vi "stimulate_and_record.vi"(3 "SSH password":string, 4 "Transfer and Run Date Folder After Experiment":bool, 5 "SSH user name":string, 6 "Tags":string, 7 "Frames":i32, 8 "Convert Power to Voltage":bool, 9 "voltages/power":dbl[](array[numeric]), 10 "parameters":string[](array[string]), 11 "parameters headers":string[](array[string])) -> ()   [LabVIEW 2014]
uses:
  <vilib>/userdefined/High Color/IMAQdx.ctl
  <vilib>/Utility/file.llb/Write To Spreadsheet File (string).vi
  <vilib>/Utility/file.llb/Read From Spreadsheet File (string).vi
  <vilib>/Utility/file.llb/Write To Spreadsheet File (DBL).vi
panel:
  out "Error":string
  out "Save Directory":path
  out "Buffer Number Out":u32
  out "Image":T1(plugin-control)
  in  "stop":bool
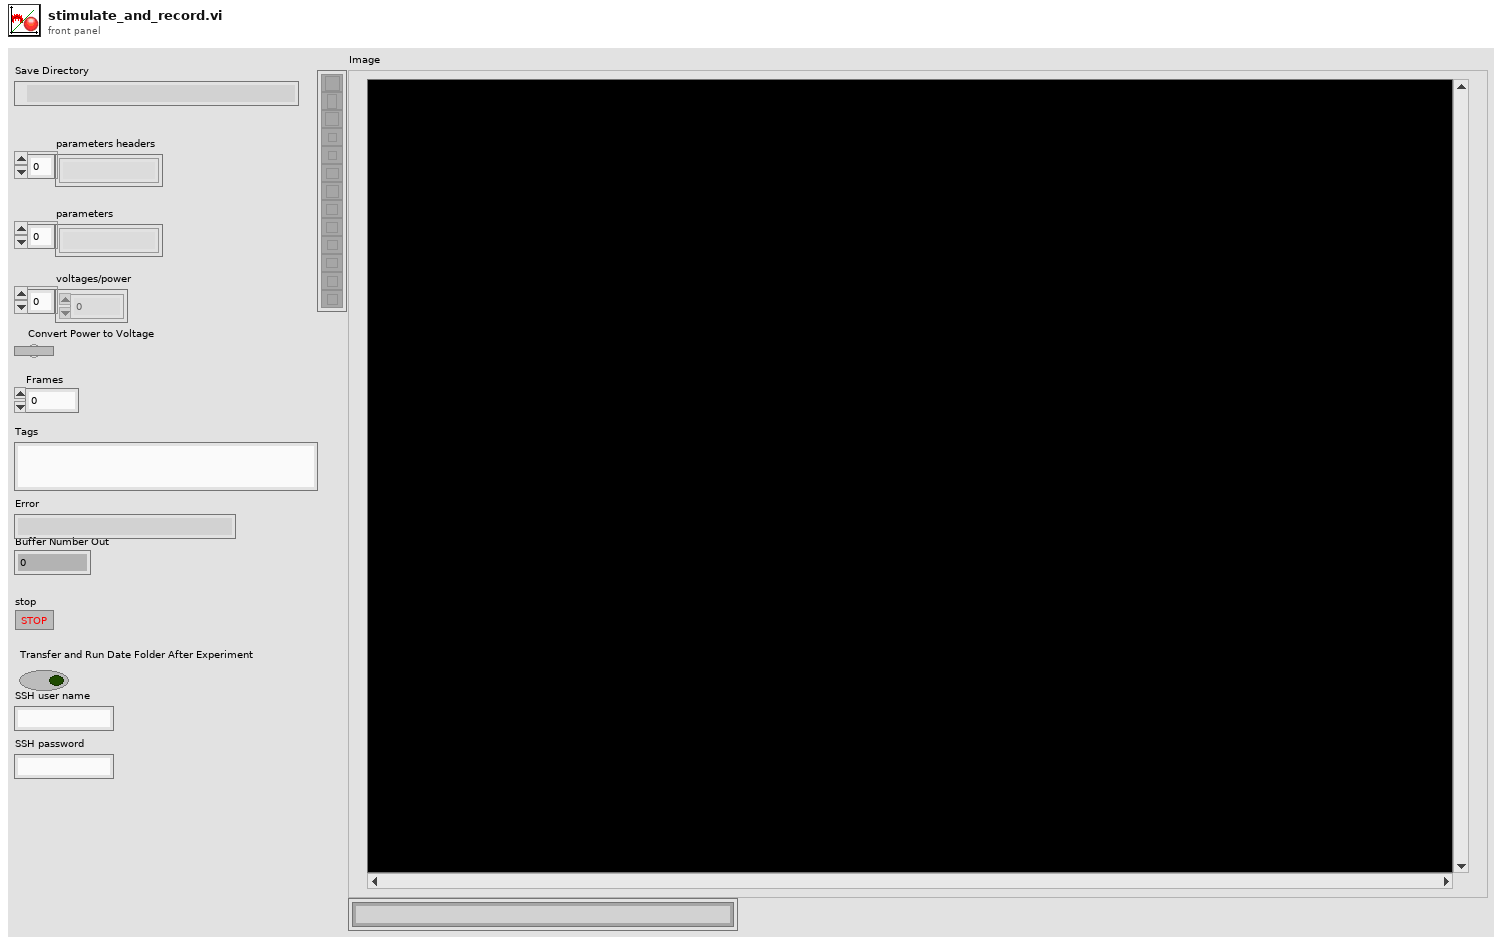
[diagram p1: front panel]
types:
  T1 = typedef "IMAQ Image.ctl" = refnum<image>
  T2 = typedef "IMAQdx.ctl" = refnum<k21>
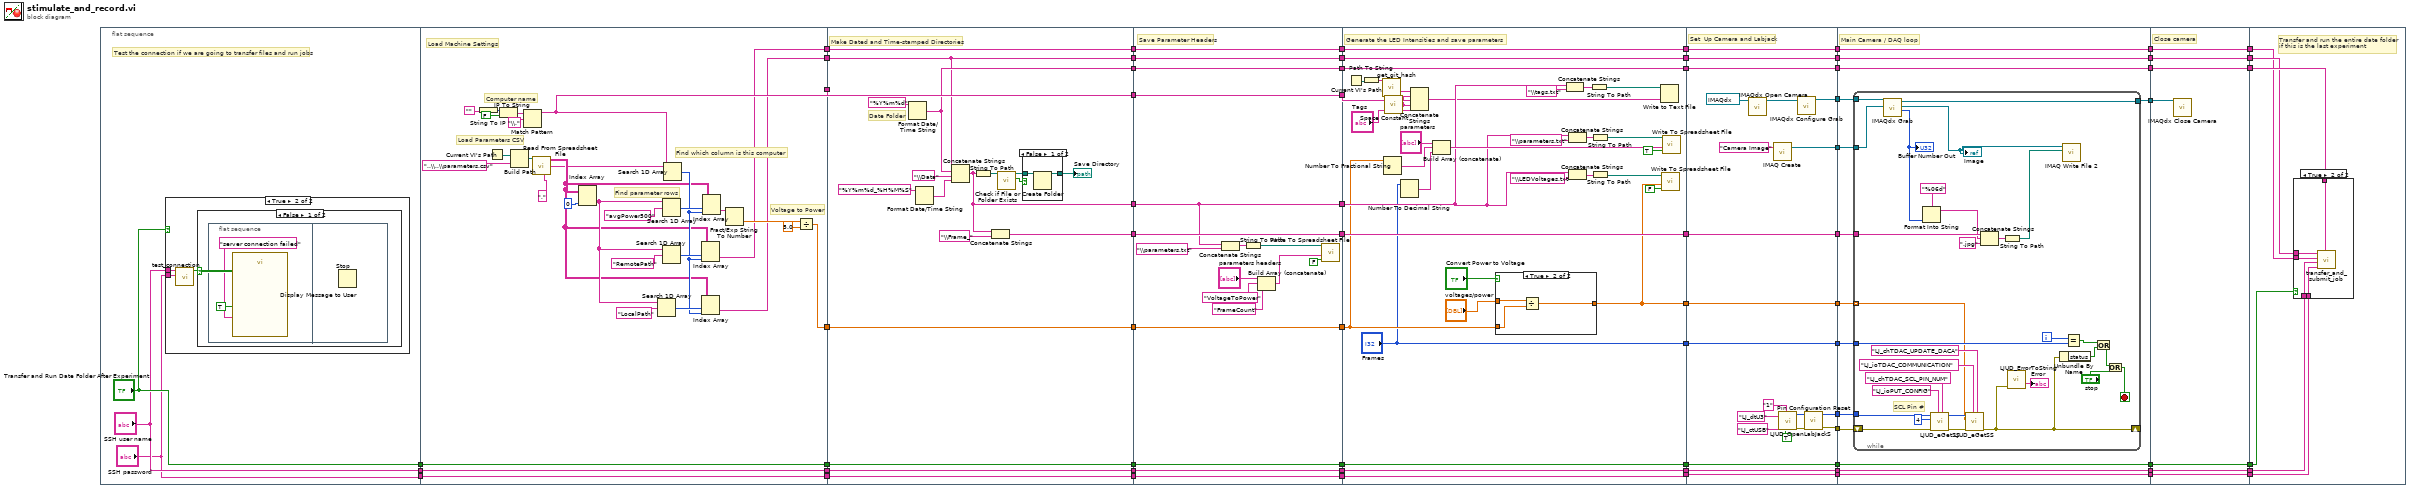
[diagram p0: block diagram]
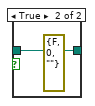
[diagram p4: hidden frame]
diagram:
  n1 = flat-sequence {
    tunnel: ["Transfer and Run Date Folder After Experiment"] -> w24
    tunnel: ["SSH user name"] -> w23
    tunnel: ["SSH password"] -> w22
    tunnel: [w95] -> w54
    tunnel: [w94] -> w53
    tunnel: [w83] -> w44
    tunnel: [w82] -> w43
    tunnel: w24 -> [w76]
    tunnel: w23 -> [w75]
    tunnel: w22 -> [w74]
    tunnel: [w76] -> w15
    tunnel: [w75] -> w8
    tunnel: [w74] -> w7
    tunnel: [w122] -> w38
    tunnel: [w121] -> w36
    tunnel: [w120] -> w34
    tunnel: [w119] -> w32
    tunnel: [w118] -> w30
    tunnel: [w117] -> w28
    tunnel: [w116] -> w26
    tunnel: w43 -> [w116]
    tunnel: w44 -> [w117]
    tunnel: w53 -> [w119]
    tunnel: w54 -> [w120]
    tunnel: [w106] -> w16
    tunnel: w15 -> [w106]
    tunnel: [w105] -> w9
    tunnel: w8 -> [w105]
    tunnel: w7 -> [w104]
    tunnel: [w104] -> w6
    tunnel: w38 -> [w143]
    tunnel: [w143] -> w37
    tunnel: w36 -> [w129]
    tunnel: [w129] -> w35
    tunnel: w34 -> [w142]
    tunnel: [w142] -> w33
    tunnel: w32 -> [w141]
    tunnel: [w141] -> w31
    tunnel: w30 -> [w140]
    tunnel: [w140] -> w29
    tunnel: w28 -> [w139]
    tunnel: [w139] -> w27
    tunnel: w26 -> [w138]
    tunnel: [w138] -> w25
    tunnel: [w128] -> w17
    tunnel: w16 -> [w128]
    tunnel: [w127] -> w10
    tunnel: w9 -> [w127]
    tunnel: w6 -> [w126]
    tunnel: [w126] -> w5
    tunnel: w37 -> [w176]
    tunnel: [w176] -> w59
    tunnel: [w156] -> w57
    tunnel: ["Frames"] -> w56
    tunnel: w35 -> [w168]
    tunnel: w33 -> [w152]
    tunnel: w31 -> [w164]
    tunnel: w29 -> [w161]
    tunnel: [w161] -> w49
    tunnel: [w160] -> w45
    tunnel: w27 -> [w160]
    tunnel: [w159] -> w39
    tunnel: w25 -> [w159]
    tunnel: [w150] -> w18
    tunnel: w17 -> [w150]
    tunnel: [w149] -> w11
    tunnel: w10 -> [w149]
    tunnel: w5 -> [w148]
    tunnel: [w148] -> w4
    tunnel: w59 -> [w199]
    tunnel: [w201] -> w65
    tunnel: [w200] -> w64
    tunnel: [w199] -> w63
    tunnel: [w191] -> w61
    tunnel: [w190] -> w60
    tunnel: [w195] -> w58
    tunnel: w57 -> [w195]
    tunnel: w56 -> [w194]
    tunnel: [w194] -> w55
    tunnel: [w188] -> w50
    tunnel: w49 -> [w188]
    tunnel: [w187] -> w46
    tunnel: w45 -> [w187]
    tunnel: [w186] -> w40
    tunnel: w39 -> [w186]
    tunnel: [w185] -> w19
    tunnel: w18 -> [w185]
    tunnel: [w184] -> w12
    tunnel: w11 -> [w184]
    tunnel: w4 -> [w183]
    tunnel: [w183] -> w3
    tunnel: w65 -> [w218]
    tunnel: w64 -> [w217]
    tunnel: w63 -> [w216]
    tunnel: [w215] -> w62
    tunnel: w61 -> [w214]
    tunnel: w60 -> [w213]
    tunnel: w58 -> [w212]
    tunnel: w55 -> [w211]
    tunnel: [w210] -> w51
    tunnel: w50 -> [w210]
    tunnel: [w209] -> w47
    tunnel: w46 -> [w209]
    tunnel: [w208] -> w41
    tunnel: w40 -> [w208]
    tunnel: [w207] -> w20
    tunnel: w19 -> [w207]
    tunnel: [w206] -> w13
    tunnel: w12 -> [w206]
    tunnel: w3 -> [w205]
    tunnel: [w205] -> w2
    tunnel: w62 -> [w255]
    tunnel: [w254] -> w52
    tunnel: w51 -> [w254]
    tunnel: [w253] -> w48
    tunnel: w47 -> [w253]
    tunnel: [w252] -> w42
    tunnel: w41 -> [w252]
    tunnel: [w251] -> w21
    tunnel: w20 -> [w251]
    tunnel: [w250] -> w14
    tunnel: w13 -> [w250]
    tunnel: w2 -> [w249]
    tunnel: [w249] -> w1
    tunnel: w52 -> [w261]
    tunnel: w48 -> [w260]
    tunnel: w42 -> [w259]
    tunnel: w21 -> [w258]
    tunnel: w14 -> [w257]
    tunnel: w1 -> [w256]
    frame #0 {
      # "Test the connection if we are going to transfer files and run jobs"
      n2 = case shown="True" "Transfer and Run Date Folder After Experiment" {
        tunnel: "SSH password" -> [_ w71]
        tunnel: "SSH user name" -> [_ w69]
        frame False {
        }
        frame True {
          n3 = call "test_connection.vi"("Username"=w69, "Password"=w71) -> ("Connection Successful"=w70:bool)  [unwired: 7 in]
          n4 = case shown="False" w70 {
            frame False {
              n5 = flat-sequence {
                frame #0 {
                  n6 = call "Display Message to User"("Enable"=TRUE, "Message"="server connection failed") -> ()  [unwired: 8 in, 2 out]
                }
                frame #1 {
                  n7 = Stop() -> ()  [unwired: 1 in]
                }
              }
            }
            frame True {
            }
          }
        }
      }
    }
    frame #1 {
      # "Find parameter rows"
      # "Find which column is this computer"
      # "Voltage to Power"
      # "Load Parameters CSV"
      # "Computer name"
      # "Load Machine Settings"
      n8 = String To IP(1:"") -> (0:w103:u32)
      n9 = Current VI's Path() -> (path=w98:path)
      n10 = IP To String(1:FALSE, 2:w103) -> (0:w100:string)
      n11 = Build Path(base path=w98, name or relative path="..\\..\\parameters.csv") -> (appended path=w80:path)
      n12 = Match Pattern(string=w100, regular expression="\\.") -> (before substring=w94:string)  [unwired: 1 in, 3 out]
      n13 = call-poly <vilib>:"Read From Spreadsheet File.vi"("delimiter (\\t)"=",", "file path (dialog if empty)"=w80) -> ("first row"=w78:string[], "all rows"=w79:string[][])  [unwired: 5 in, 3 out]
      n14 = Index Array(array=w79, index (col)=0) -> (element=w81:string[])  [unwired: 1 in]
      n15 = Search 1D Array(1D array=w81, element="LocalPath") -> (index of element=w85:i32)  [unwired: 1 in]
      n16 = Search 1D Array(1D array=w81, element="RemotePath") -> (index of element=w89:i32)  [unwired: 1 in]
      n17 = Search 1D Array(1D array=w81, element="avgPower500") -> (index of element=w90:i32)  [unwired: 1 in]
      n18 = Search 1D Array(1D array=w78, element=w94) -> (index of element=w84:i32)  [unwired: 1 in]
      n19 = Index Array(array=w79, index (row)=w89, index (col)=w84) -> (element=w82:string)
      n20 = Index Array(array=w79, index (row)=w85, index (col)=w84) -> (element=w83:string)
      n21 = Index Array(array=w79, index (row)=w90, index (col)=w84) -> (element=w88:string)
      n22 = Fract/Exp String To Number(string=w88) -> (number=w87:dbl)  [unwired: 3 in, 1 out]
      n23 = Divide(x=w87, y=5.0) -> (x/y=w95:dbl)
    }
    frame #2 {
      # "Date Folder"
      # "Make Dated and Time-stamped Directories"
      n24 = Format Date/Time String(time format string (%c)="%Y%m%d") -> (date/time string=w118:string)  [unwired: 2 in]
      n25 = Format Date/Time String(time format string (%c)="%Y%m%d_%H%M%S") -> (date/time string=w110:string)  [unwired: 2 in]
      n26 = Concatenate Strings(w117, w118, "\\Data", w110) -> (w121:string)
      n27 = String To Path(string=w121) -> (path=w109:path)
      n28 = Concatenate Strings(w121, "\\Frame_") -> (w122:string)
      n29 = call <vilib>:"Check if File or Folder Exists.vi"("path"=w109) -> ("file or folder exists?"=w114:bool, "dup path"=w113:path)  [unwired: 8 in, 1 out]
      n30 = case shown="False" w114 {
        tunnel: [w123 w125] -> w108
        tunnel: w113 -> [w124 w125]
        frame False {
          n31 = Create Folder(path (use dialog)=w124) -> (created path=w123:path)  [unwired: 2 in, 2 out]
        }
        frame True {
          (unwired) errorcluster {"status"=FALSE, "code"=0, "source"=""} ("error out")
        }
      }
      "Save Directory" <- w108
    }
    frame #3 {
      # "Save Parameter Headers"
      n32 = Concatenate Strings(w129, "\\parameters.txt") -> (w137:string)
      n33 = String To Path(string=w137) -> (path=w136:path)
      n34 = Build Array (concatenate)("parameters headers", "VoltageToPower", "FrameCount") -> (w133:string[])
      n35 = call-poly <vilib>:"Write To Spreadsheet File.vi"("append to file? (new file:F)"=FALSE, "1D data"=w133, "file path (dialog if empty)"=w136) -> ()  [unwired: 5 in, 1 out]
    }
    frame #4 {
      # "Generate the LED Intensities and save parameters"
      n36 = Current VI's Path() -> (path=w146:path)
      n37 = Path To String(path=w146) -> (string=w147:string)
      n38 = call "get_git_hash.vi"("VI folder"=w147) -> ("github hash"=w144:string)  [unwired: 10 in]
      n39 = Number To Fractional String(number=w152) -> (F-format string=w153:string)  [unwired: 3 in]
      n40 = call <vilib>:"Space Constant.vi"() -> ("String"=w145:string)
      n41 = Number To Decimal String(number="Frames") -> (decimal integer string=w154:string)  [unwired: 1 in]
      n42 = Concatenate Strings(w144, w145, w164, w145, "Tags") -> (w162:string)
      n43 = Build Array (concatenate)("parameters", w153, w154) -> (w169:string[])
      n44 = case shown="True" "Convert Power to Voltage" {
        tunnel: "voltages/power" -> [w179 w182]
        tunnel: [w179 w180] -> w156
        tunnel: w152 -> [_ w181]
        frame False {
        }
        frame True {
          n45 = Divide(x=w182, y=w181) -> (x/y=w180:dbl[])
        }
      }
      n46 = Concatenate Strings(w168, "\\tags.txt") -> (w166:string)
      n47 = Concatenate Strings(w168, "\\LEDVoltages.txt") -> (w178:string)
      n48 = Concatenate Strings(w168, "\\parameters.txt") -> (w173:string)
      n49 = String To Path(string=w166) -> (path=w165:path)
      n50 = String To Path(string=w178) -> (path=w177:path)
      n51 = String To Path(string=w173) -> (path=w172:path)
      n52 = Write to Text File(file (use dialog)=w165, text=w162) -> ()  [unwired: 2 in, 3 out]
      n53 = call-poly <vilib>:"Write To Spreadsheet File.vi"("append to file? (new file:F)"=FALSE, "1D data"=w156, "file path (dialog if empty)"=w177) -> ()  [unwired: 5 in, 1 out]
      n54 = call-poly <vilib>:"Write To Spreadsheet File.vi"("append to file? (new file:F)"=TRUE, "1D data"=w169, "file path (dialog if empty)"=w172) -> ()  [unwired: 5 in, 1 out]
    }
    frame #5 {
      # "Set  Up Camera and Labjack"
      n55 = call <vilib>:"IMAQdx Open Camera.vi"("Session In"=T2 "cam0") -> ("Session Out"=w203:T2)  [unwired: 9 in, 1 out]
      n56 = call "IMAQ Create"("Image Name"="Camera Image") -> ("New Image"=w200:T1)  [unwired: 4 in, 1 out]
      n57 = call "LJUD_OpenLabJackS.vi"("FirstFound"=TRUE, "Address"="1" ("DeviceType"), "ConnectionType"="LJ_ctUSB", "DeviceType"="LJ_dtU3") -> ("error out"=w189:errorcluster, "Handle"=w192:i32)  [unwired: 5 in, 1 out]
      n58 = call <vilib>:"IMAQdx Configure Grab.vi"("Session In"=w203) -> ("Session Out"=w201:T2)  [unwired: 9 in, 1 out]
      n59 = call "Pin Configuration Reset.vi"("error in"=w189, "Handle In"=w192) -> ("error out"=w190:errorcluster, "Handle Out"=w191:i32)  [unwired: 8 in]
    }
    frame #6 {
      # "Main Camera / DAQ loop"
      n60 = while {
        tunnel: w218 -> [w248]
        tunnel: [w247] -> w215
        tunnel: w217 -> [w246]
        tunnel: w216 -> [w244]
        tunnel: w214 -> [w221]
        shift-right: [w222] -> _
        shift-left: w213 -> [w220]
        tunnel: w212 -> [w219] mode=indexing
        tunnel: w211 -> [w230]
        i -> [w231]
        stop <- w237 stop-if-true
        # "SCL Pin #"
        n61 = call <vilib>:"IMAQdx Grab.vi"("Image In"=w246, "Session In"=w248) -> ("Buffer Number Out"=w240:u32, "Image Out"=w245:T1, "Session Out"=w247:T2)  [unwired: 6 in, 1 out]
        "Image" <- w245
        "Buffer Number Out" <- w240
        n62 = Format Into String(format string="%06d" ("string"), w240) -> (resulting string=w239:string)  [unwired: 2 in, 1 out]
        n63 = call "LJUD_eGetSS.vi"("Channel"="LJ_chTDAC_SCL_PIN_NUM", "IOType"="LJ_ioPUT_CONFIG", "error in"=w220, "Value Write"=4, "Handle In"=w221) -> ("error out"=w223:errorcluster, "Handle Out"=w226:i32)  [unwired: 4 in, 1 out]
        n64 = call "LJUD_eGetSS.vi"("Channel"="LJ_chTDAC_UPDATE_DACA", "IOType"="LJ_ioTDAC_COMMUNICATION", "error in"=w223, "Value Write"=w219, "Handle In"=w226) -> ("error out"=w222:errorcluster)  [unwired: 4 in, 2 out]
        n65 = Concatenate Strings(w244, w239, ".jpg" ("string")) -> (w242:string)
        n66 = String To Path(string=w242) -> (path=w241:path)
        n67 = call "LJUD_ErrorToString.vi"("error in"=w222) -> ("String"=→"Error":string)  [unwired: 10 in]
        n68 = Unbundle By Name(w222) -> ("status"=w234:bool)
        n69 = call-poly "IMAQ Write File 2"("File Path"=w241, "Image"=w245) -> ()  [unwired: 8 in, 2 out]
        n70 = Equal?(x=w231, y=w230) -> (x = y?=w233:bool)
        n71 = Or(x=w233, y=w234) -> (x .or. y?=w232:bool)
        n72 = Or(x=w232, y="stop") -> (x .or. y?=w237:bool)
      }
    }
    frame #7 {
      # "Close camera"
      n73 = call <vilib>:"IMAQdx Close Camera.vi"("Session In"=w255) -> ()  [unwired: 10 in, 1 out]
    }
    frame #8 {
      # "Transfer and run the entire date folder\nif this is the last experiment"
      n74 = case shown="True" w258 {
        tunnel: w261 -> [_ w266]
        tunnel: w260 -> [_ w265]
        tunnel: w259 -> [_ w264]
        tunnel: w257 -> [_ w263]
        tunnel: w256 -> [_ w262]
        frame False {
        }
        frame True {
          n75 = call "transfer_and_submit_job.vi"("Date Folder"=w266, "Password"=w262, "Username"=w263, "Remote Data Directory"=w264, "Local Data Directory"=w265) -> ()  [unwired: 7 in]
        }
      }
    }
  }
